vi "Eval Condition.vi"(7 "Variables":refnum<class "Variables.lvclass">, 8 "error in (no error)":errorcluster, 9 "Sequence Time":T1, 11 "SeqLoaded Condition in":refnum<class "SeqLoaded Condition.lvclass">) -> (0 "error out":errorcluster, 2 "Result":bool, 3 "SeqLoaded Condition out":refnum<class "SeqLoaded Condition.lvclass">)   [LabVIEW 2020, in "VolatusSeq.lvlib" / "SeqLoaded Condition.lvclass"]
uses:
  SeqLoaded Condition.lvclass
  SeqLoaded Condition.lvclass/SeqLoaded Condition.ctl
  Volatus/MessageQ/MessageQ.lvclass
  Sequence Status Value/Sequence Status Value.lvclass
  Variables/Variables.lvclass
  Sequence Time.ctl
  VolatusSeq.lvlib
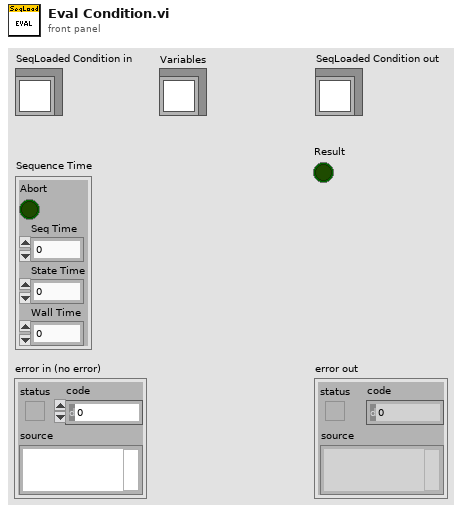
[diagram p1: front panel]
types:
  T1 = typedef "VolatusSeq.lvlib/Sequence Time.ctl" = cluster{"Abort":bool, "Seq Time":dbl, "State Time":dbl, "Wall Time":dbl}
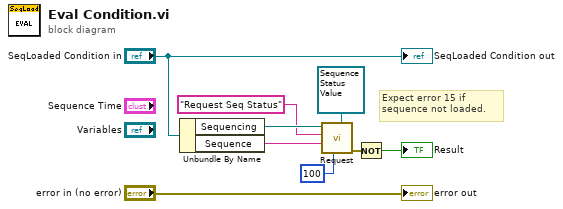
[diagram p0: block diagram]
diagram:
  # "Expect error 15 if sequence not loaded."
  n1 = Unbundle By Name("SeqLoaded Condition in") -> ("Sequencing"=w7:refnum<class "MessageQ.lvclass">, "Sequence"=w5:string)
  n2 = call "Request.vi"("Response Type (None)"=refnum<class "Sequence Status Value.lvclass"> refnum ("VolatusSeq.lvlib:Sequence Status Value.lvclass"), "Timeout ms (1000)"=100, "Data"=w5, "ID"="Request Seq Status", "MessageQ in"=w7) -> ("error out"=w2:errorcluster)  [unwired: 4 in, 2 out]
  n3 = Not(x=w2) -> (.not. x?=→"Result":bool)
  "error out" <- "error in (no error)"
  "SeqLoaded Condition out" <- "SeqLoaded Condition in"
